vi "Get Connection Reference (Serial).vi"(8 "error in":errorcluster, 11 "connection info in":T1) -> (0 "error out":errorcluster, 2 "VISA resource name out":refnum<visa-resource-name>, 3 "connection info out":T1)   [LabVIEW 2013, in "NI STM.lvlib"]
doc: "Returns the serial VISA reference."
uses:
  NI STM.lvlib
  Serial Connection Info.ctl
  SubVIs/MetaDataElement.ctl
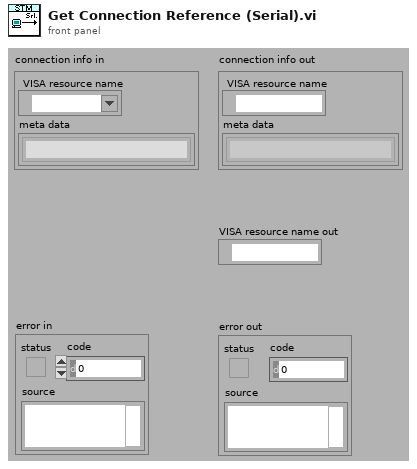
[diagram p1: front panel]
types:
  T1 = typedef "NI STM.lvlib/Serial Connection Info.ctl" = cluster{"VISA resource name":refnum<visa-resource-name>, "meta data":T2[]}
  T2 = typedef "NI STM.lvlib/MetaDataElement.ctl" = string
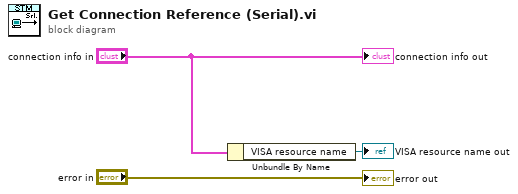
[diagram p0: block diagram]
diagram:
  n1 = Unbundle By Name("connection info in") -> ("VISA resource name"=→"VISA resource name out":refnum<visa-resource-name>)
  "connection info out" <- "connection info in"
  "error out" <- "error in"
